vi "Set Sensor Servo.vi"(6 "sensor servo error (0)":i32, 8 "error in (no error)":errorcluster, 10 "sensor servo":refnum<class "NI_Robotics_Starter Kit Servo Motor.lvclass">, 11 "NI_Robotics_Starter Kit Host in":refnum<class "NI_Robotics_Starter Kit Host.lvclass">) -> (0 "error out":errorcluster, 3 "NI_Robotics_Starter Kit Host out":refnum<class "NI_Robotics_Starter Kit Host.lvclass">)   [LabVIEW 2017, in "NI_Robotics_Starter Kit Host.lvclass"]
uses:
  <vilib>/robotics/Starter Kit/Host Interface/NI_Robotics_Starter Kit Host.lvclass
  <vilib>/robotics/Starter Kit/Servo Motor/NI_Robotics_Starter Kit Servo Motor.lvclass
  <vilib>/robotics/Starter Kit/Host Interface/NI_Robotics_Starter Kit Host.lvclass/NI_Robotics_Starter Kit Host.ctl
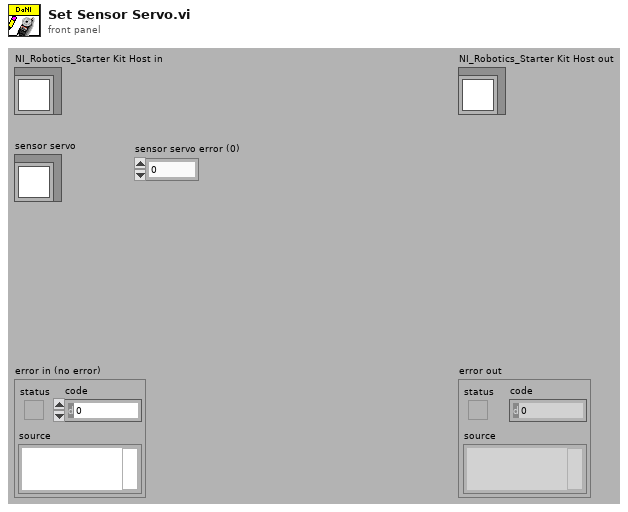
[diagram p1: front panel]
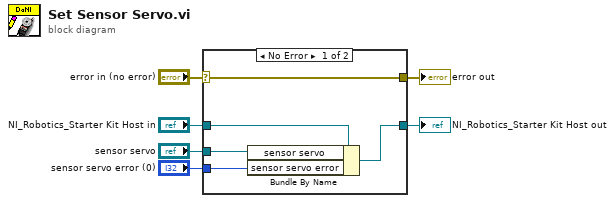
[diagram p0: block diagram]
diagram:
  n1 = case shown="No Error" "error in (no error)" {
    selector: "error in (no error)" -> [w11 w12]
    tunnel: [w11 w12] -> w5
    tunnel: [w9 w13] -> w3
    tunnel: "NI_Robotics_Starter Kit Host in" -> [w10 w13]
    tunnel: "sensor servo" -> [w8 _]
    tunnel: "sensor servo error (0)" -> [w7 _]
    frame No Error {
      n2 = Bundle By Name(cluster=w10, "sensor servo"=w8, "sensor servo error"=w7) -> (w9:refnum<class "NI_Robotics_Starter Kit Host.lvclass">)
    }
    frame Error {
    }
  }
  "error out" <- w5
  "NI_Robotics_Starter Kit Host out" <- w3
